vi "FGV FT-IR Diagnosewerte.vi"(6 "Aktionen":T4, 8 "FT-IR MAX":T2, 9 "FT-IR MIN":T3, 10 "Zykluszeit ToolWeb":u32, 11 "Diagnose neu":T1) -> (0 "FT-IR MAX":T2, 1 "FT-IR MIN":T3, 2 "Druck":dbl, 3 "Temperatur":dbl, 4 "Diagnose mean":T1, 5 "Diagnose":T1)   [LabVIEW 2020, in "FT-IR.lvlib"]
uses:
  FT-IR.lvlib
  FGV FT-IR Diagnose Aktionen.ctl
  TOOLweb Interface Library/TOOLweb Diagnose.ctl
  <vilib>/Analysis/baseanly.llb/Mean (DBL).vi
  <vilib>/Analysis/NI_AALBase.lvlib
  Messdaten/Messdaten.lvlib
  TOOLweb Interface Library/Typdefinitionen.lvlib
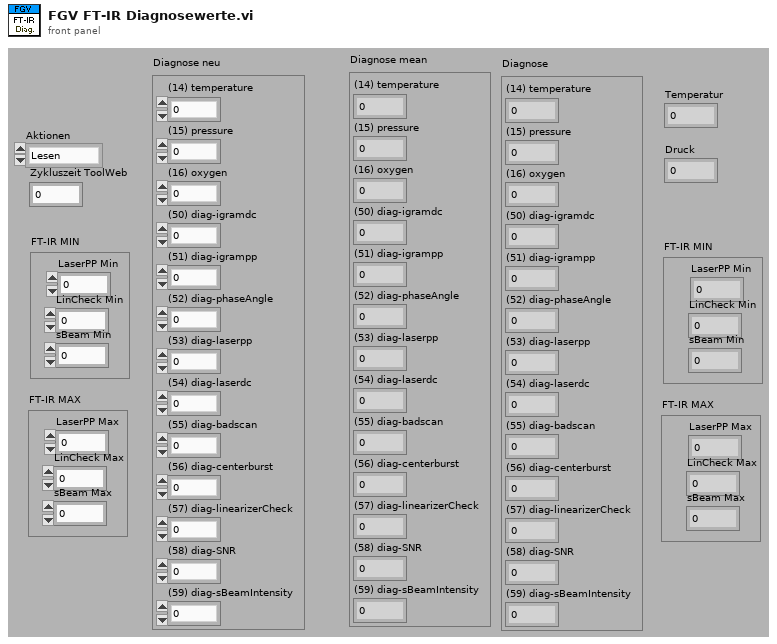
[diagram p1: front panel]
types:
  T1 = typedef "FT-IR.lvlib/TOOLweb Interface.lvlib/Typdefinitionen.lvlib/TOOLweb Diagnose.ctl" = cluster{"(14) temperature":sgl, "(15) pressure":sgl, "(16) oxygen":sgl, "(50) diag-igramdc":sgl, "(51) diag-igrampp":sgl, "(52) diag-phaseAngle":sgl, "(53) diag-laserpp":sgl, "(54) diag-laserdc":sgl, "(55) diag-badscan":sgl, "(56) diag-centerburst":sgl, "(57) diag-linearizerCheck":sgl, "(58) diag-SNR":sgl, "(59) diag-sBeamIntensity":sgl}
  T2 = cluster{"LaserPP Max":dbl, "LinCheck Max":dbl, "sBeam Max":dbl}
  T3 = cluster{"LaserPP Min":dbl, "LinCheck Min":dbl, "sBeam Min":dbl}
  T4 = typedef "FT-IR.lvlib/FGV FT-IR Diagnose Aktionen.ctl" = enum16{"Lesen", "Diagnose Schreiben", "Min Schreiben", "Max Schreiben"}
  T5 = cluster{"[0]":dbl, "[1]":dbl, "[2]":dbl, "[3]":dbl, "[4]":dbl, "[5]":dbl, "[6]":dbl, "[7]":dbl, "[8]":dbl, "[9]":dbl, "[10]":dbl, "[11]":dbl, "[12]":dbl}
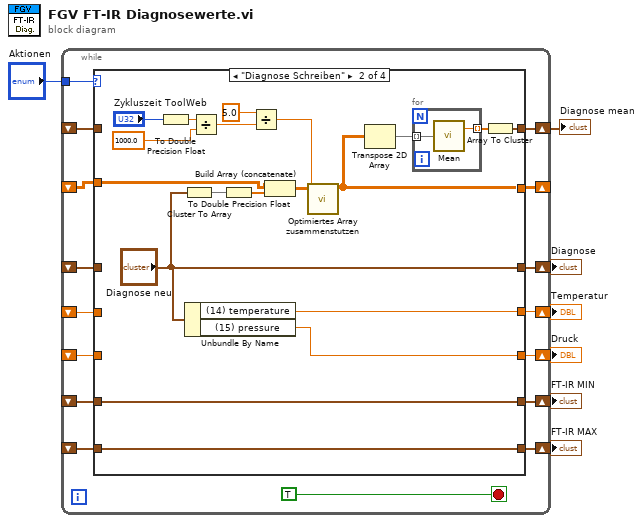
[diagram p0: block diagram]
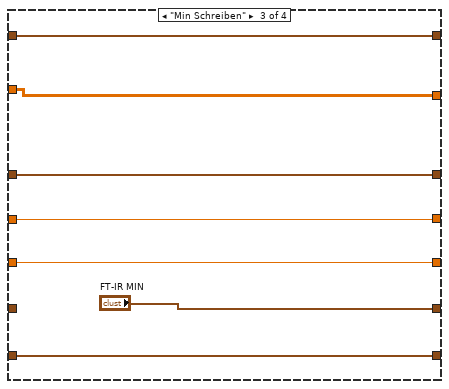
[diagram p3: hidden frame]
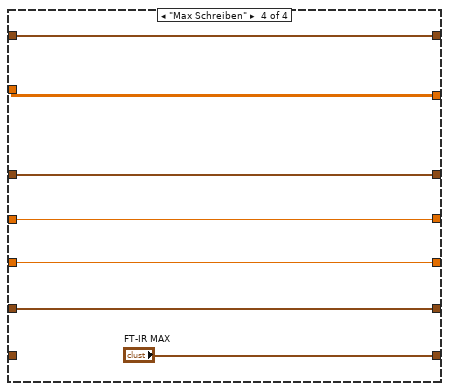
[diagram p4: hidden frame]
diagram:
  n1 = while {
    tunnel: "Aktionen" -> [w22]
    shift-right: [w21] -> w6
    shift-left: _ -> [w20]
    shift-right: [w19] -> w5
    shift-left: _ -> [w17]
    shift-right: [w18] -> w4
    shift-left: _ -> [w16]
    shift-right: [w15] -> w3
    shift-left: _ -> [w12]
    shift-right: [w13] -> w2
    shift-left: _ -> [w14]
    shift-right: [w11] -> _
    shift-left: _ -> [w10]
    shift-right: [w9] -> w1
    shift-left: _ -> [w8]
    stop <- TRUE stop-if-true
    n2 = case shown="\"Diagnose Schreiben\"" w22 {
      tunnel: [w30 "Diagnose neu" w56 w64] -> w21
      tunnel: w20 -> [w30 _ w56 w64]
      tunnel: [w29 w49 w57 w63] -> w19
      tunnel: [w28 w48 w55 w62] -> w18
      tunnel: w17 -> [w29 _ w57 w63]
      tunnel: w16 -> [w28 _ w55 w62]
      tunnel: [w27 w47 "FT-IR MIN" w61] -> w15
      tunnel: [w26 w46 w54 "FT-IR MAX"] -> w13
      tunnel: w14 -> [w26 w46 w54 _]
      tunnel: w12 -> [w27 w47 _ w61]
      tunnel: [w24 w31 w53 w59] -> w11
      tunnel: w10 -> [w24 w37 w53 w59]
      tunnel: [w25 w34 w52 w60] -> w9
      tunnel: w8 -> [w25 _ w52 w60]
      frame "Lesen", Default {
      }
      frame "Diagnose Schreiben" {
        n3 = To Double Precision Float(number="Zykluszeit ToolWeb") -> (double precision float=w43:dbl)
        n4 = Cluster To Array(cluster="Diagnose neu") -> (array=w39:sgl[])
        n5 = Unbundle By Name("Diagnose neu") -> ("(14) temperature"=w49:sgl, "(15) pressure"=w48:sgl)
        n6 = Divide(x=w43, y=1000.0) -> (x/y=w44:dbl)
        n7 = To Double Precision Float(number=w39) -> (double precision float=w38:dbl[])
        n8 = Divide(x=5.0, y=w44) -> (x/y=w32:dbl)
        n9 = Build Array (concatenate)(w37, w38) -> (w33:dbl[][])
        n10 = call "Optimiertes Array zusammenstutzen.vi"("Anzahl Elemente"=w32, "Messdaten"=w33) -> ("Messdaten"=w31:sgl[][])  [unwired: 8 in, 1 out]
        n11 = Transpose 2D Array(2D array=w31) -> (transposed array=w36:sgl[][])
        n12 = for {
          tunnel: w36 -> [w50] mode=indexing
          tunnel: [w51] -> w35 mode=indexing
          n13 = call-poly <vilib>:"Mean.vi"("X"=w50) -> ("mean"=w51:dbl)  [unwired: 1 out]
        }
        n14 = Array To Cluster(array=w35) -> (cluster=w34:T5)
      }
      frame "Min Schreiben" {
      }
      frame "Max Schreiben" {
      }
    }
  }
  "Diagnose" <- w6
  "Temperatur" <- w5
  "Druck" <- w4
  "FT-IR MIN" <- w3
  "FT-IR MAX" <- w2
  "Diagnose mean" <- w1
